vi "Calculate Color Index Array.vi"(8 "error in (no error)":errorcluster, 10 "3D Mesh Datatype in":refnum<class "3D Mesh Datatype.lvclass">, 11 "Plot Representation In":T1) -> (0 "error out":errorcluster, 2 "3D Mesh Datatype out":refnum<class "3D Mesh Datatype.lvclass">, 3 "Plot Representation Out":T1)   [LabVIEW 2020, in "3D Mesh Datatype.lvclass"]
uses:
  <vilib>/Math Plots/3D Math Plots/3D Mesh/3D Mesh Datatype/3D Mesh Datatype.lvclass
  <vilib>/Math Plots/3D Math Plots/3D Plot/3D Plot/Typedef/Plot Representation.ctl
  <vilib>/Math Plots/3D Math Plots/3D Plot/3D Plot/Typedef/Range Clusters.ctl
  <vilib>/Math Plots/3D Math Plots/3D Plot/3D Plot/Typedef/Mesh Data.ctl
  <vilib>/Math Plots/3D Math Plots/3D Mesh/3D Mesh Datatype/3D Mesh Datatype.lvclass/3D Mesh Datatype.ctl
  <vilib>/Math Plots/3D Math Plots/3D Plot/3D Plot Datatype/3D Plot Datatype.lvclass
  <vilib>/Math Plots/3D Math Plots/3D Plot/3D Plot/3D Plot.lvclass
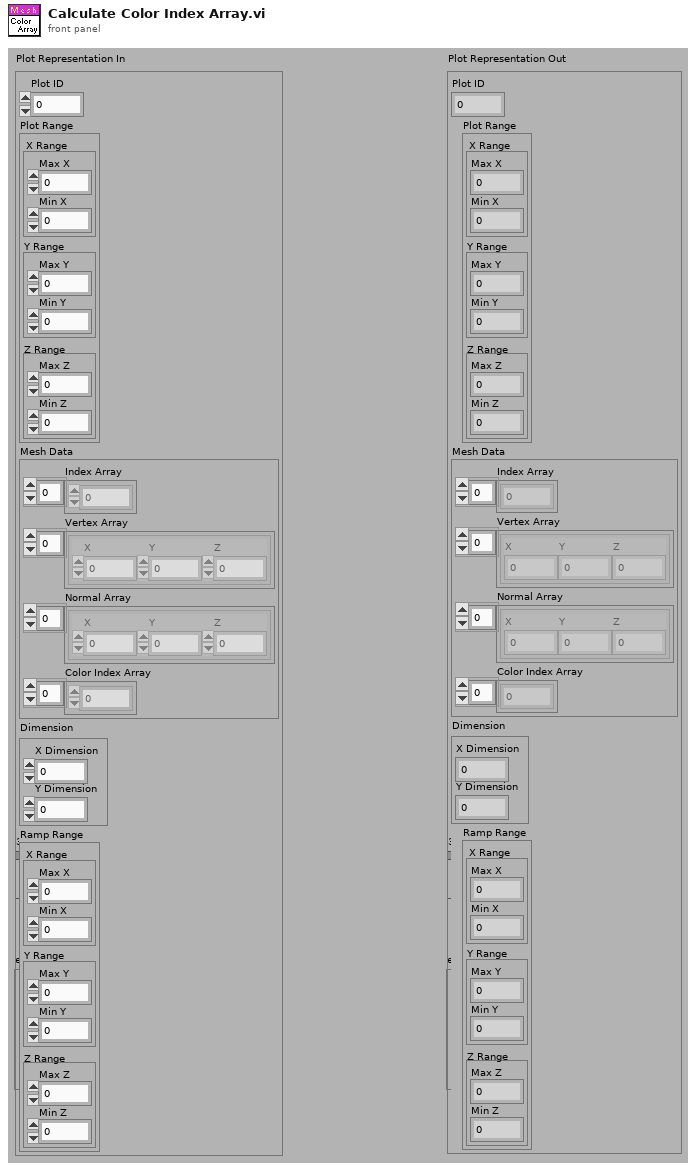
[diagram p1: front panel]
types:
  T1 = typedef "3D Plot.lvclass/Plot Representation.ctl" = cluster{"Plot ID":i32, "Plot Range":T2, "Mesh Data":T3, "Dimension":cluster{"X Dimension":i32, "Y Dimension":i32}, "Ramp Range":T2}
  T2 = typedef "3D Plot.lvclass/Range Clusters.ctl" = cluster{"X Range":cluster{"Max X":sgl, "Min X":sgl}, "Y Range":cluster{"Max Y":sgl, "Min Y":sgl}, "Z Range":cluster{"Max Z":sgl, "Min Z":sgl}}
  T3 = typedef "3D Plot.lvclass/Mesh Data.ctl" = cluster{"Index Array":u32[], "Vertex Array":cluster{"X":sgl, "Y":sgl, "Z":sgl}[], "Normal Array":cluster{"X":sgl, "Y":sgl, "Z":sgl}[], "Color Index Array":i32[]}
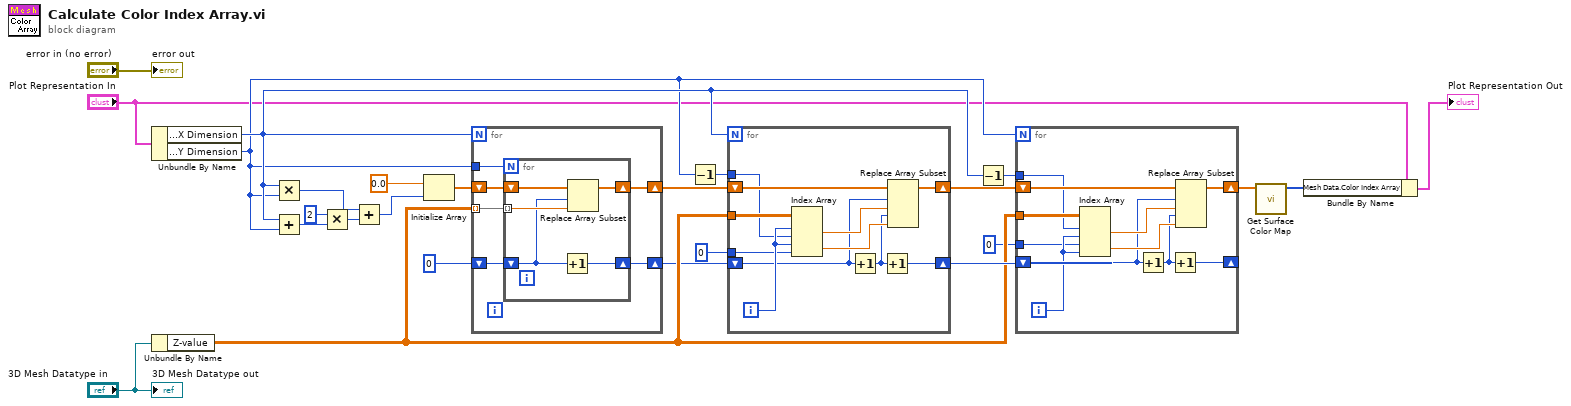
[diagram p0: block diagram]
diagram:
  n1 = Unbundle By Name("Plot Representation In") -> ("Dimension.X Dimension"=w9:i32, "Dimension.Y Dimension"=w8:i32)
  n2 = Unbundle By Name("3D Mesh Datatype in") -> ("Z-value"=w6:sgl[][])
  n3 = Multiply(x=w9, y=w8) -> (x*y=w11:i32)
  n4 = Add(x=w9, y=w8) -> (x+y=w13:i32)
  n5 = Multiply(x=2, y=w13) -> (x*y=w12:i32)
  n6 = Add(x=w11, y=w12) -> (x+y=w10:i32)
  n7 = Initialize Array(sgl 0.0 ("element"), w10) -> (w21:sgl[])
  n8 = for {
    N: w9 -> [_]
    tunnel: w8 -> [w31]
    shift-right: [w26] -> w7
    shift-left: w21 -> [w30]
    tunnel: w6 -> [w29] mode=indexing
    shift-right: [w28] -> w2
    shift-left: 0 -> [w27]
    n9 = for {
      N: w31 -> [_]
      shift-right: [w35] -> w26
      shift-left: w30 -> [w36]
      tunnel: w29 -> [w34] mode=indexing
      shift-right: [w33] -> w28
      shift-left: w27 -> [w32]
      n10 = Increment(x=w32) -> (x+1=w33:i32)
      n11 = Replace Array Subset(array=w36, new element=w34, index=w32) -> (w35:sgl[])
    }
  }
  n12 = Decrement(x=w8) -> (x-1=w16:i32)
  n13 = for {
    N: w9 -> [_]
    shift-right: [w45] -> w15
    shift-left: w7 -> [w46]
    tunnel: w6 -> [w47]
    tunnel: w16 -> [w43]
    tunnel: 0 -> [w42]
    shift-right: [w39] -> w18
    shift-left: w2 -> [w37]
    i -> [w44]
    n14 = Index Array(array=w47, index (row) #1=w44, index (col) #1=w43, index (row) #2=w44, index (col) #2=w42) -> (element #1=w40:sgl, element #2=w41:sgl)
    n15 = Increment(x=w37) -> (x+1=w38:i32)
    n16 = Increment(x=w38) -> (x+1=w39:i32)
    n17 = Replace Array Subset(array=w46, new element #1=w40, index #1=w37, new element #2=w41, index #2=w38) -> (w45:sgl[])
  }
  n18 = Decrement(x=w9) -> (x-1=w17:i32)
  n19 = for {
    N: w8 -> [_]
    shift-right: [w56] -> w3
    shift-left: w15 -> [w57]
    tunnel: w6 -> [w58]
    tunnel: w17 -> [w54]
    tunnel: 0 -> [w53]
    shift-right: [w50] -> _
    shift-left: w18 -> [w48]
    i -> [w55]
    n20 = Index Array(array=w58, index (row) #1=w54, index (col) #1=w55, index (row) #2=w53, index (col) #2=w55) -> (element #1=w51:sgl, element #2=w52:sgl)
    n21 = Increment(x=w48) -> (x+1=w49:i32)
    n22 = Increment(x=w49) -> (x+1=w50:i32)
    n23 = Replace Array Subset(array=w57, new element #1=w51, index #1=w48, new element #2=w52, index #2=w49) -> (w56:sgl[])
  }
  n24 = call <vilib>:"Get Surface Color Map.vi"("Amplifiy"=w3) -> ("Color Index Array"=w23:i32[])  [unwired: 1 in, 9 out]
  n25 = Bundle By Name(cluster="Plot Representation In", "Mesh Data.Color Index Array"=w23) -> (→"Plot Representation Out":T1)
  "error out" <- "error in (no error)"
  "3D Mesh Datatype out" <- "3D Mesh Datatype in"
